vi "ReadTMXfile.vi"(8 "error in (no error)":errorcluster, 10 "path to tmx-file (created with Tiles2D)":path=path "/home/lvuser/natinst/bin/data/maps/Menu.tmx") -> (0 "error out":errorcluster, 2 "Tilenumbers":u32[][](array[numeric]))   [LabVIEW 2019, in "RT_Game.lvlib" / "Game.lvclass"]
uses:
  Game.lvclass
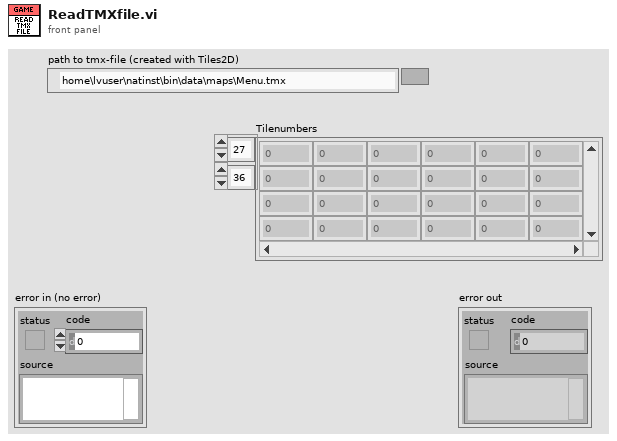
[diagram p1: front panel]
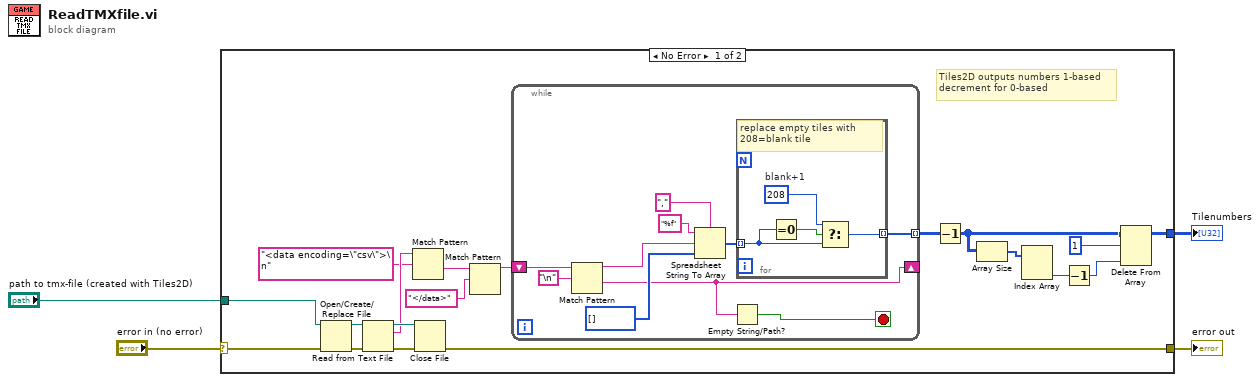
[diagram p0: block diagram]
diagram:
  n1 = case shown="No Error" "error in (no error)" {
    selector: "error in (no error)" -> [w23 w38]
    tunnel: [w20 w38] -> w3
    tunnel: "path to tmx-file (created with Tiles2D)" -> [w17 _]
    tunnel: [w10 _] -> w1
    frame No Error {
      # "Tiles2D outputs numbers 1-based\ndecrement for 0-based"
      n2 = Open/Create/Replace File(file path (use dialog)=w17, error in=w23) -> (refnum out=w19:refnum<file>, error out=w22:errorcluster)  [unwired: 4 in, 1 out]
      n3 = Read from Text File(file (use dialog)=w19, error in=w22) -> (refnum out=w18:refnum<file>, text=w16:string, error out=w21:errorcluster)  [unwired: 2 in, 1 out]
      n4 = Match Pattern(string=w16, regular expression="<data encoding=\"csv\">\n") -> (after substring=w13:string)  [unwired: 1 in, 3 out]
      n5 = Close File(refnum=w18, error in=w21) -> (error out=w20:errorcluster)  [unwired: 1 out]
      n6 = Match Pattern(string=w13, regular expression="</data>") -> (before substring=w12:string)  [unwired: 1 in, 3 out]
      n7 = while {
        tunnel: [w28] -> w11 mode=indexing
        shift-right: [w24] -> _
        shift-left: w12 -> [w26]
        stop <- w27 stop-if-true
        n8 = Match Pattern(string=w26, regular expression="\n") -> (before substring=w25:string, after substring=w24:string)  [unwired: 1 in, 2 out]
        n9 = Spreadsheet String To Array(delimiter (Tab)=",", format string="%f", spreadsheet string=w25, array type (2D Dbl)=u32[] []) -> (array=w29:u32[])
        n10 = Empty String/Path?(string/path=w24) -> (empty?=w27:bool)
        n11 = for {
          tunnel: w29 -> [w37] mode=indexing
          tunnel: [w36] -> w28 mode=indexing
          w34 = u32 208  # blank+1
          # "replace empty tiles with\n208=blank tile"
          n12 = Equal To 0?(x=w37) -> (x = 0?=w35:bool)
          n13 = Select(t=w34, s=w35, f=w37) -> (s? t:f=w36:u32)
        }
      }
      n14 = Decrement(x=w11) -> (x-1=w8:u32[][])
      n15 = Array Size(array=w8) -> (size(s)=w7:i32[])
      n16 = Index Array(array=w7) -> (element #2=w6:i32)  [unwired: 2 in, 1 out]
      n17 = Decrement(x=w6) -> (x-1=w5:i32)
      n18 = Delete From Array(array=w8, length=1, index (col)=w5) -> (array with subset deleted=w10:u32[][])  [unwired: 1 in, 1 out]
    }
    frame Error {
    }
  }
  "error out" <- w3
  "Tilenumbers" <- w1
